vi "Generate HW Config XML.vi"() -> ()   [LabVIEW 2017]
panel:
  in  "Rx Start Channel":i32
  in  "Tx Start Channel":i32
  in  "file path (use dialog)":path
  in  "Core ID":i32=-1
  in  "Core Name":string="CoreName"
  in  "Number of Tx Channels":i32
  in  "Messages per Tx Channel":i32
  in  "Number of Rx Channels":i32
  in  "Labels per Rx Channel":i32
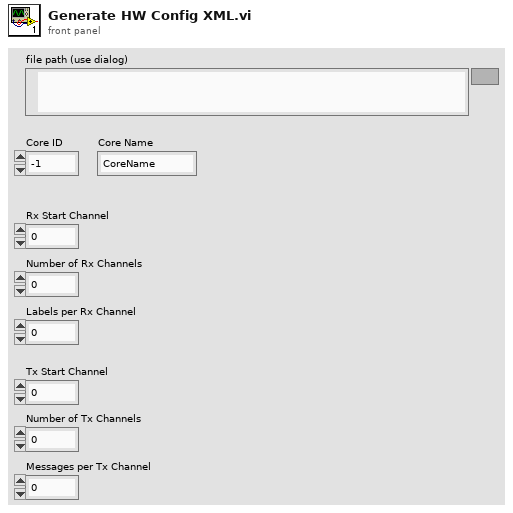
[diagram p1: front panel]
types:
  T1 = enum16{"open", "replace", "create", "open or create", "replace or create", "replace or create with confirmation"}
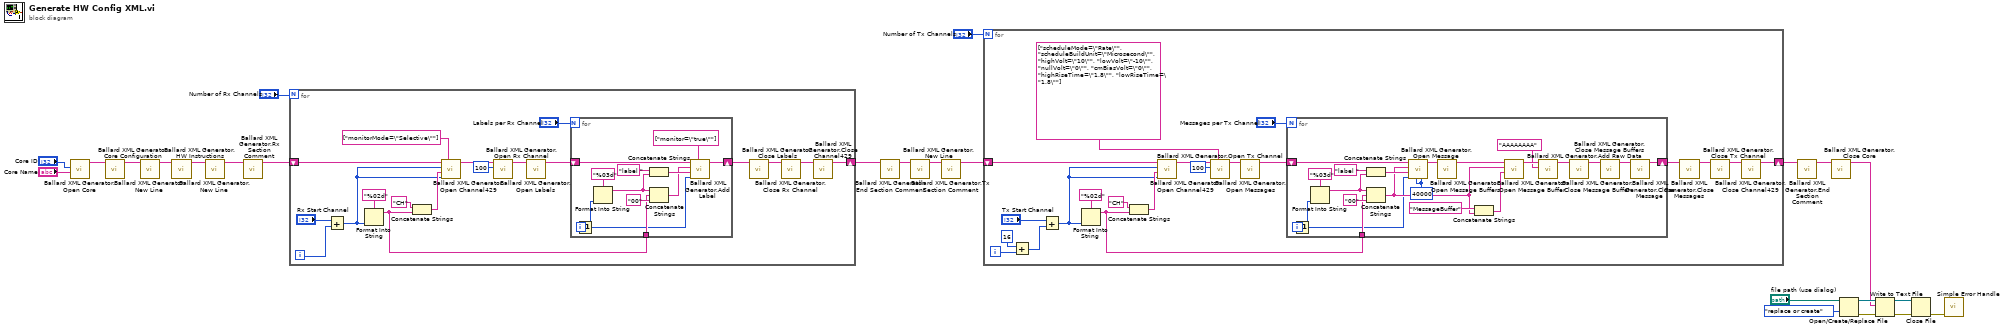
[diagram p0: block diagram]
diagram:
  n1 = call "Ballard XML Generator.Open Core.vi"("name"="Core Name", "id"="Core ID") -> ("string out"=w24:string)  [unwired: 9 in]
  n2 = call "Ballard XML Generator.Core Configuration.vi"("string in"=w24) -> ("string out"=w23:string)  [unwired: 10 in]
  n3 = call "Ballard XML Generator.New Line.vi"("string in"=w23) -> ("string out"=w22:string)  [unwired: 10 in]
  n4 = call "Ballard XML Generator.HW Instructions.vi"("string in"=w22) -> ("string out"=w21:string)  [unwired: 10 in]
  n5 = call "Ballard XML Generator.New Line.vi"("string in"=w21) -> ("string out"=w20:string)  [unwired: 10 in]
  n6 = call "Ballard XML Generator.Rx Section Comment.vi"("string in"=w20) -> ("string out"=w19:string)  [unwired: 10 in]
  n7 = for {
    N: "Number of Rx Channels" -> [_]
    shift-right: [w28] -> w16
    shift-left: w19 -> [w42]
    i -> [w27]
    n8 = Add(x="Rx Start Channel", y=w27) -> (x+y=w26:i32)
    n9 = Format Into String(format string="%02d", w26) -> (resulting string=w29:string)  [unwired: 2 in, 1 out]
    n10 = Concatenate Strings("CH" ("string"), w29) -> (w31:string)
    n11 = call "Ballard XML Generator.Open Channel429.vi"("other params"=string[] ["monitorMode=\"Selective\""], "hardware channel"=w26, "name"=w31, "id"=w26, "string in"=w42) -> ("string out"=w41:string)  [unwired: 6 in]
    n12 = call "Ballard XML Generator.Open Rx Channel.vi"("speedKHz"=100, "string in"=w41) -> ("string out"=w38:string)  [unwired: 9 in]
    n13 = call "Ballard XML Generator.Open Labels.vi"("string in"=w38) -> ("string out"=w37:string)  [unwired: 10 in]
    n14 = for {
      N: "Labels per Rx Channel" -> [_]
      shift-right: [w52] -> w36
      shift-left: w37 -> [w54]
      tunnel: w29 -> [w49]
      i -> [w44]
      n15 = Increment(x=w44) -> (x+1=w43:i32)
      n16 = Format Into String(format string="%03d", w43) -> (resulting string=w47:string)  [unwired: 2 in, 1 out]
      n17 = Concatenate Strings("label ", w47) -> (w46:string)
      n18 = Concatenate Strings(w47, w49, "00" ("string")) -> (w45:string)
      n19 = call "Ballard XML Generator.Add Label.vi"("other params"=string[] ["monitor=\"true\""], "label decimal"=w43, "name"=w46, "id"=w45, "string in"=w54) -> ("string out"=w52:string)  [unwired: 6 in]
    }
    n20 = call "Ballard XML Generator.Close Labels.vi"("string in"=w36) -> ("string out"=w35:string)  [unwired: 10 in]
    n21 = call "Ballard XML Generator.Close Rx Channel.vi"("string in"=w35) -> ("string out"=w34:string)  [unwired: 10 in]
    n22 = call "Ballard XML Generator.Close Channel429.vi"("string in"=w34) -> ("string out"=w28:string)  [unwired: 10 in]
  }
  n23 = call "Ballard XML Generator.End Section Comment.vi"("string in"=w16) -> ("string out"=w15:string)  [unwired: 10 in]
  n24 = call "Ballard XML Generator.New Line.vi"("string in"=w15) -> ("string out"=w14:string)  [unwired: 10 in]
  n25 = call "Ballard XML Generator.Tx Section Comment.vi"("string in"=w14) -> ("string out"=w13:string)  [unwired: 10 in]
  n26 = for {
    N: "Number of Tx Channels" -> [_]
    shift-right: [w67] -> w12
    shift-left: w13 -> [w74]
    i -> [w69]
    n27 = Add(x=16, y=w69) -> (x+y=w57:i32)
    n28 = Add(x="Tx Start Channel", y=w57) -> (x+y=w56:i32)
    n29 = Format Into String(format string="%02d", w56) -> (resulting string=w68:string)  [unwired: 2 in, 1 out]
    n30 = Concatenate Strings("CH" ("string"), w68) -> (w71:string)
    n31 = call "Ballard XML Generator.Open Channel429.vi"("hardware channel"=w56, "name"=w71, "id"=w56, "string in"=w74) -> ("string out"=w65:string)  [unwired: 7 in]
    n32 = call "Ballard XML Generator.Open Tx Channel.vi"("other params"=string[] ["scheduleMode=\"Rate\"", "scheduleBuildUnit=\"Microsecond\"", "highVolt=\"10\"", "lowVolt=\"-10\"", "nullVolt=\"0\"", "cmBiasVolt=\"0\"", "highRiseTime=\"1.8\"", "lowRiseTime=\"1.8\""], "speedKHz"=100, "string in"=w65) -> ("string out"=w62:string)  [unwired: 8 in]
    n33 = call "Ballard XML Generator.Open Messages.vi"("string in"=w62) -> ("string out"=w61:string)  [unwired: 10 in]
    n34 = for {
      N: "Messages per Tx Channel" -> [_]
      shift-right: [w80] -> w60
      shift-left: w61 -> [w95]
      tunnel: w68 -> [w92]
      i -> [w88]
      w76 = 40000 ("minRate (400)")
      n35 = Increment(x=w88) -> (x+1=w75:i32)
      n36 = Format Into String(format string="%03d", w75) -> (resulting string=w90:string)  [unwired: 2 in, 1 out]
      n37 = Concatenate Strings("label ", w90) -> (w89:string)
      n38 = Concatenate Strings(w90, w92, "00" ("string")) -> (w78:string)
      n39 = call "Ballard XML Generator.Open Message.vi"("minRate (400)"=w76, "maxRate (400)"=w76, "labelDecimal"=w75, "name"=w89, "id"=w78, "string in"=w95) -> ("string out"=w87:string)  [unwired: 5 in]
      n40 = call "Ballard XML Generator.Open Message Buffers.vi"("string in"=w87) -> ("string out"=w86:string)  [unwired: 10 in]
      n41 = Concatenate Strings("MessageBuffer" ("name"), w78) -> (w77:string)
      n42 = call "Ballard XML Generator.Open Message Buffer.vi"("name"=w77, "id"=w78, "string in"=w86) -> ("string out"=w85:string)  [unwired: 8 in]
      n43 = call "Ballard XML Generator.Add Raw Data.vi"("raw data"="AAAAAAAA", "string in"=w85) -> ("string out"=w83:string)  [unwired: 9 in]
      n44 = call "Ballard XML Generator.Close Message Buffer.vi"("string in"=w83) -> ("string out"=w82:string)  [unwired: 10 in]
      n45 = call "Ballard XML Generator.Close Message Buffers.vi"("string in"=w82) -> ("string out"=w81:string)  [unwired: 10 in]
      n46 = call "Ballard XML Generator.Close Message.vi"("string in"=w81) -> ("string out"=w80:string)  [unwired: 10 in]
    }
    n47 = call "Ballard XML Generator.Close Messages.vi"("string in"=w60) -> ("string out"=w59:string)  [unwired: 10 in]
    n48 = call "Ballard XML Generator.Close Tx Channel.vi"("string in"=w59) -> ("string out"=w58:string)  [unwired: 10 in]
    n49 = call "Ballard XML Generator.Close Channel429.vi"("string in"=w58) -> ("string out"=w67:string)  [unwired: 10 in]
  }
  n50 = call "Ballard XML Generator.End Section Comment.vi"("string in"=w12) -> ("string out"=w11:string)  [unwired: 10 in]
  n51 = call "Ballard XML Generator.Close Core.vi"("string in"=w11) -> ("string out"=w1:string)  [unwired: 10 in]
  n52 = Open/Create/Replace File(file path (use dialog)="file path (use dialog)", operation (0:open)=T1."replace or create") -> (refnum out=w6:refnum<file>, error out=w5:errorcluster)  [unwired: 4 in, 1 out]
  n53 = Write to Text File(file (use dialog)=w6, text=w1, error in=w5) -> (refnum out=w4:refnum<file>, error out=w3:errorcluster)  [unwired: 1 in, 1 out]
  n54 = Close File(refnum=w4, error in=w3) -> (error out=w2:errorcluster)  [unwired: 1 out]
  n55 = call <vilib>:"Simple Error Handler.vi"("error in (no error)"=w2) -> ()  [unwired: 4 in, 5 out]
